vi "set DIO0 out.vi"(8 "error in":errorcluster) -> (0 "error out":errorcluster)   [LabVIEW 2024]
uses:
  <vilib>/rvi/Emulation/niFpgaGetClockAttributes.vi
  <vilib>/rvi/Emulation/niFpgaSctlEmulationGetInTimedLoop.vi
  <vilib>/rvi/Emulation/niFpgaEmulationReportErrorSimple.vi
  <vilib>/rvi/eio/common/nirviEmuTemplateMethod_errors.vi
  <vilib>/rvi/Emulation/niFpgaCriticalErrorInLSC.vi
  <vilib>/eio/EIOMethodNode/EIOMethodNode.xnode
  <vilib>/eio/EIONode/EIONode.xnode
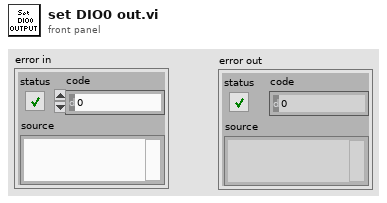
[diagram p1: front panel]
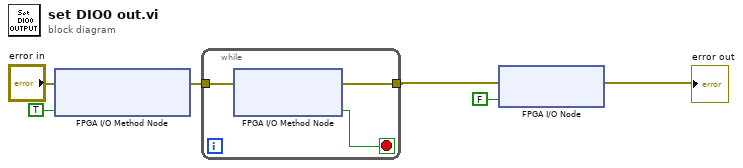
[diagram p0: block diagram]
diagram:
  n1 = xnode "FPGA I/O Method Node"("error in"="error in", "Enable"=TRUE) -> ("error out"=w6:errorcluster)  [unwired: 1 in, 1 out]
  n2 = while {
    tunnel: w6 -> [w9]
    tunnel: [w8] -> w2
    stop <- w7 stop-if-true
    n3 = xnode "FPGA I/O Method Node"("error in"=w9) -> ("error out"=w8:errorcluster, "Ready"=w7:bool)  [unwired: 1 in, 1 out]
  }
  n4 = xnode "FPGA I/O Node"("error in"=w2, "Mod2/DIO0"=FALSE) -> ("error out"=→"error out":errorcluster)  [unwired: 1 in, 1 out]
